vi "H2O und CO2 Werte.vi"(9 "CO2 Index":i32, 10 "H2O Index":i32, 11 "Mittelwertdaten":sgl[][](array[numeric])) -> (2 "CO2 Wert":sgl, 3 "H2O Wert":sgl)   [LabVIEW 2020, in "FT-IR.lvlib"]
uses:
  FT-IR.lvlib
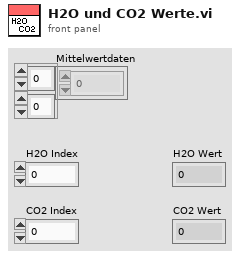
[diagram p1: front panel]
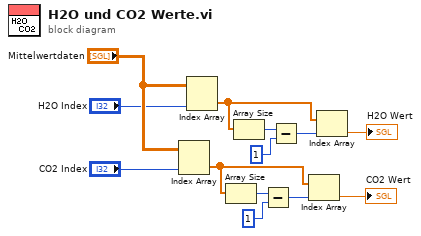
[diagram p0: block diagram]
diagram:
  n1 = Index Array(array="Mittelwertdaten", index (col)="CO2 Index") -> (element=w6:sgl[])  [unwired: 1 in]
  n2 = Index Array(array="Mittelwertdaten", index (col)="H2O Index") -> (element=w2:sgl[])  [unwired: 1 in]
  n3 = Array Size(array=w6) -> (size(s)=w7:i32)
  n4 = Array Size(array=w2) -> (size(s)=w3:i32)
  n5 = Subtract(x=w7, y=1) -> (x-y=w10:i32)
  n6 = Subtract(x=w3, y=1) -> (x-y=w11:i32)
  n7 = Index Array(array=w6, index=w10) -> (element=→"CO2 Wert":sgl)
  n8 = Index Array(array=w2, index=w11) -> (element=→"H2O Wert":sgl)
